vi "Main.vi"(7 "sweep rate, /min":dbl=0.2, 8 "sweep to:":dbl=-0.5, 9 "sweep":T6(radio)=enum."time_sweep") -> ()   [LabVIEW 2017] (continued)
                          tunnel: w749 -> [w752 w758]
                          tunnel: [w752 w757] -> w748
                          tunnel: w747 -> [w751 w755]
                          tunnel: [w751 w753] -> w746
                          frame False {
                            # "not measure 2182A 1 channel 1 (2182A_1_ch1)"
                          }
                          frame True {
                            w754 = "2182A_1_ch1"
                            # "measure 2182A 1 channel 1 (2182A_1_ch1)"
                            n675 = local read "2182A 1 addr"() -> (w759:u8)
                            n676 = Number To Decimal String(number=w759) -> (decimal integer string=w760:string)  [unwired: 1 in]
                            n677 = GPIB Clear(3:w760) -> ()  [unwired: 1 in, 2 out]
                            n678 = Build Array (concatenate)(w755, w754) -> (w753:string[])
                            n679 = Concatenate Strings(w758, w754, "\t") -> (w757:string)
                          }
                        }
                        n680 = property on="Figure_axis" class="Arr (strict)"("Value"=w746) -> ()  [unwired: 2 in, 2 out]
                        n681 = property on="data_caption" class="Str"("Value"=w748) -> ()  [unwired: 2 in, 2 out]
                      }
                      frame #27 {
                        # "2182A 1 channel 2 measure (2182A_1_ch2)"
                        n682 = local read "2182A 1 ch2"() -> (w765:bool)
                        n683 = property on="Figure_axis" class="Arr (strict)"() -> ("Value"=w762:string[])  [unwired: 2 in, 2 out]
                        n684 = property on="data_caption" class="Str"() -> ("Value"=w764:string)  [unwired: 2 in, 2 out]
                        n685 = case shown="True" w765 {
                          tunnel: w764 -> [w767 w773]
                          tunnel: [w767 w772] -> w763
                          tunnel: w762 -> [w766 w770]
                          tunnel: [w766 w768] -> w761
                          frame False {
                            # "not measure 2182A 1 channel 2 (2182A_1_ch2)"
                          }
                          frame True {
                            w769 = "2182A_1_ch2"
                            # "measure 2182A 1 channel 2 (2182A_1_ch2)"
                            n686 = local read "2182A 1 addr"() -> (w774:u8)
                            n687 = Number To Decimal String(number=w774) -> (decimal integer string=w775:string)  [unwired: 1 in]
                            n688 = GPIB Clear(3:w775) -> ()  [unwired: 1 in, 2 out]
                            n689 = Build Array (concatenate)(w770, w769) -> (w768:string[])
                            n690 = Concatenate Strings(w773, w769, "\t") -> (w772:string)
                          }
                        }
                        n691 = property on="Figure_axis" class="Arr (strict)"("Value"=w761) -> ()  [unwired: 2 in, 2 out]
                        n692 = property on="data_caption" class="Str"("Value"=w763) -> ()  [unwired: 2 in, 2 out]
                      }
                      frame #28 {
                        # "2182A 2 channel 1 measure (2182A_2_ch1)"
                        n693 = local read "2182A 2 ch1"() -> (w780:bool)
                        n694 = property on="Figure_axis" class="Arr (strict)"() -> ("Value"=w777:string[])  [unwired: 2 in, 2 out]
                        n695 = property on="data_caption" class="Str"() -> ("Value"=w779:string)  [unwired: 2 in, 2 out]
                        n696 = case shown="True" w780 {
                          tunnel: w779 -> [w782 w788]
                          tunnel: [w782 w787] -> w778
                          tunnel: w777 -> [w781 w785]
                          tunnel: [w781 w783] -> w776
                          frame False {
                            # "not measure 2182A 2 channel 1 (2182A_2_ch1)"
                          }
                          frame True {
                            w784 = "2182A_2_ch1"
                            # "measure 2182A 2 channel 1 (2182A_2_ch1)"
                            n697 = local read "2182A 2 addr"() -> (w789:u8)
                            n698 = Number To Decimal String(number=w789) -> (decimal integer string=w790:string)  [unwired: 1 in]
                            n699 = GPIB Clear(3:w790) -> ()  [unwired: 1 in, 2 out]
                            n700 = Build Array (concatenate)(w785, w784) -> (w783:string[])
                            n701 = Concatenate Strings(w788, w784, "\t") -> (w787:string)
                          }
                        }
                        n702 = property on="Figure_axis" class="Arr (strict)"("Value"=w776) -> ()  [unwired: 2 in, 2 out]
                        n703 = property on="data_caption" class="Str"("Value"=w778) -> ()  [unwired: 2 in, 2 out]
                      }
                      frame #29 {
                        # "2182A 2 channel 2 measure (2182A_2_ch2)"
                        n704 = local read "2182A 2 ch2"() -> (w795:bool)
                        n705 = property on="Figure_axis" class="Arr (strict)"() -> ("Value"=w792:string[])  [unwired: 2 in, 2 out]
                        n706 = property on="data_caption" class="Str"() -> ("Value"=w794:string)  [unwired: 2 in, 2 out]
                        n707 = case shown="True" w795 {
                          tunnel: w794 -> [w797 w803]
                          tunnel: [w797 w802] -> w793
                          tunnel: w792 -> [w796 w800]
                          tunnel: [w796 w798] -> w791
                          frame False {
                            # "not measure 2182A 2 channel 2 (2182A_2_ch2)"
                          }
                          frame True {
                            w799 = "2182A_2_ch2"
                            # "measure 2182A 2 channel 2 (2182A_2_ch2)"
                            n708 = local read "2182A 2 addr"() -> (w804:u8)
                            n709 = Number To Decimal String(number=w804) -> (decimal integer string=w805:string)  [unwired: 1 in]
                            n710 = GPIB Clear(3:w805) -> ()  [unwired: 1 in, 2 out]
                            n711 = Build Array (concatenate)(w800, w799) -> (w798:string[])
                            n712 = Concatenate Strings(w803, w799, "\t") -> (w802:string)
                          }
                        }
                        n713 = property on="Figure_axis" class="Arr (strict)"("Value"=w791) -> ()  [unwired: 2 in, 2 out]
                        n714 = property on="data_caption" class="Str"("Value"=w793) -> ()  [unwired: 2 in, 2 out]
                      }
                      frame #30 {
                        # "2182A 3 channel 1 measure (2182A_3_ch1)"
                        n715 = local read "2182A 3 ch1"() -> (w810:bool)
                        n716 = property on="Figure_axis" class="Arr (strict)"() -> ("Value"=w807:string[])  [unwired: 2 in, 2 out]
                        n717 = property on="data_caption" class="Str"() -> ("Value"=w809:string)  [unwired: 2 in, 2 out]
                        n718 = case shown="True" w810 {
                          tunnel: w809 -> [w812 w818]
                          tunnel: [w812 w817] -> w808
                          tunnel: w807 -> [w811 w815]
                          tunnel: [w811 w813] -> w806
                          frame False {
                            # "not measure 2182A 3 channel 1 (2182A_3_ch1)"
                          }
                          frame True {
                            w814 = "2182A_3_ch1"
                            # "measure 2182A 3 channel 1 (2182A_3_ch1)"
                            n719 = local read "2182A 3 addr"() -> (w819:u8)
                            n720 = Number To Decimal String(number=w819) -> (decimal integer string=w820:string)  [unwired: 1 in]
                            n721 = GPIB Clear(3:w820) -> ()  [unwired: 1 in, 2 out]
                            n722 = Build Array (concatenate)(w815, w814) -> (w813:string[])
                            n723 = Concatenate Strings(w818, w814, "\t") -> (w817:string)
                          }
                        }
                        n724 = property on="Figure_axis" class="Arr (strict)"("Value"=w806) -> ()  [unwired: 2 in, 2 out]
                        n725 = property on="data_caption" class="Str"("Value"=w808) -> ()  [unwired: 2 in, 2 out]
                      }
                      frame #31 {
                        # "2182A 3 channel 2 measure (2182A_3_ch2)"
                        n726 = local read "2182A 3 ch2"() -> (w825:bool)
                        n727 = property on="Figure_axis" class="Arr (strict)"() -> ("Value"=w822:string[])  [unwired: 2 in, 2 out]
                        n728 = property on="data_caption" class="Str"() -> ("Value"=w824:string)  [unwired: 2 in, 2 out]
                        n729 = case shown="False" w825 {
                          tunnel: w824 -> [w827 w833]
                          tunnel: [w827 w832] -> w823
                          tunnel: w822 -> [w826 w830]
                          tunnel: [w826 w828] -> w821
                          frame False {
                            # "not measure 2182A 3 channel 2 (2182A_3_ch2)"
                          }
                          frame True {
                            w829 = "2182A_3_ch2"
                            # "measure 2182A 3 channel 2 (2182A_3_ch2)"
                            n730 = local read "2182A 3 addr"() -> (w834:u8)
                            n731 = Number To Decimal String(number=w834) -> (decimal integer string=w835:string)  [unwired: 1 in]
                            n732 = GPIB Clear(3:w835) -> ()  [unwired: 1 in, 2 out]
                            n733 = Build Array (concatenate)(w830, w829) -> (w828:string[])
                            n734 = Concatenate Strings(w833, w829, "\t") -> (w832:string)
                          }
                        }
                        n735 = property on="Figure_axis" class="Arr (strict)"("Value"=w821) -> ()  [unwired: 2 in, 2 out]
                        n736 = property on="data_caption" class="Str"("Value"=w823) -> ()  [unwired: 2 in, 2 out]
                      }
                      frame #32 {
                        # "2182A 4 channel 1 measure (2182A_4_ch1)"
                        n737 = local read "2182A 4 ch1"() -> (w840:bool)
                        n738 = property on="Figure_axis" class="Arr (strict)"() -> ("Value"=w837:string[])  [unwired: 2 in, 2 out]
                        n739 = property on="data_caption" class="Str"() -> ("Value"=w839:string)  [unwired: 2 in, 2 out]
                        n740 = case shown="True" w840 {
                          tunnel: w839 -> [w842 w848]
                          tunnel: [w842 w847] -> w838
                          tunnel: w837 -> [w841 w845]
                          tunnel: [w841 w843] -> w836
                          frame False {
                            # "not measure 2182A 4 channel 1 (2182A_4_ch1)"
                          }
                          frame True {
                            w844 = "2182A_4_ch1"
                            # "measure 2182A 4 channel 1 (2182A_4_ch1)"
                            n741 = local read "2182A 4 addr"() -> (w849:u8)
                            n742 = Number To Decimal String(number=w849) -> (decimal integer string=w850:string)  [unwired: 1 in]
                            n743 = GPIB Clear(3:w850) -> ()  [unwired: 1 in, 2 out]
                            n744 = Build Array (concatenate)(w845, w844) -> (w843:string[])
                            n745 = Concatenate Strings(w848, w844, "\t") -> (w847:string)
                          }
                        }
                        n746 = property on="Figure_axis" class="Arr (strict)"("Value"=w836) -> ()  [unwired: 2 in, 2 out]
                        n747 = property on="data_caption" class="Str"("Value"=w838) -> ()  [unwired: 2 in, 2 out]
                      }
                      frame #33 {
                        # "2182A 4 channel 2 measure (2182A_4_ch2)"
                        n748 = local read "2182A 4 ch2"() -> (w855:bool)
                        n749 = property on="Figure_axis" class="Arr (strict)"() -> ("Value"=w852:string[])  [unwired: 2 in, 2 out]
                        n750 = property on="data_caption" class="Str"() -> ("Value"=w854:string)  [unwired: 2 in, 2 out]
                        n751 = case shown="True" w855 {
                          tunnel: w854 -> [w857 w863]
                          tunnel: [w857 w862] -> w853
                          tunnel: w852 -> [w856 w860]
                          tunnel: [w856 w858] -> w851
                          frame False {
                            # "not measure 2182A 4 channel 2 (2182A_4_ch2)"
                          }
                          frame True {
                            w859 = "2182A_4_ch2"
                            # "measure 2182A 4 channel 2 (2182A_4_ch2)"
                            n752 = local read "2182A 4 addr"() -> (w864:u8)
                            n753 = Number To Decimal String(number=w864) -> (decimal integer string=w865:string)  [unwired: 1 in]
                            n754 = GPIB Clear(3:w865) -> ()  [unwired: 1 in, 2 out]
                            n755 = Build Array (concatenate)(w860, w859) -> (w858:string[])
                            n756 = Concatenate Strings(w863, w859, "\t") -> (w862:string)
                          }
                        }
                        n757 = property on="Figure_axis" class="Arr (strict)"("Value"=w851) -> ()  [unwired: 2 in, 2 out]
                        n758 = property on="data_caption" class="Str"("Value"=w853) -> ()  [unwired: 2 in, 2 out]
                      }
                      frame #34 {
                        # "2636A smua measure voltage (2636A_smua_v)"
                        n759 = local read "2636A smua meas v"() -> (w870:bool)
                        n760 = property on="Figure_axis" class="Arr (strict)"() -> ("Value"=w867:string[])  [unwired: 2 in, 2 out]
                        n761 = property on="data_caption" class="Str"() -> ("Value"=w869:string)  [unwired: 2 in, 2 out]
                        n762 = case shown="True" w870 {
                          tunnel: w869 -> [w872 w883]
                          tunnel: [w872 w882] -> w868
                          tunnel: w867 -> [w871 w880]
                          tunnel: [w871 w878] -> w866
                          frame False {
                            # "not measure voltage on 2636A smua (2636A_smua_v)"
                          }
                          frame True {
                            w879 = "2636A_smua_v"
                            # "measure voltage on 2636A smua (2636A_smua_v)"
                            n763 = local read "2336A addr"() -> (w874:refnum<visa-resource-name>)
                            n764 = VISA Open(VISA resource name=w874) -> (VISA resource name=w873:refnum<visa-resource-name>, error out=w875:errorcluster)  [unwired: 4 in]
                            n765 = VISA Clear(VISA resource name=w873, error in (no error)=w875) -> (VISA resource name out=w877:refnum<visa-resource-name>)  [unwired: 1 out]
                            n766 = property class="Instr"(reference=w877, "General Settings:Timeout Value"=u32 10000) -> ()  [unwired: 1 in, 2 out]
                            n767 = Build Array (concatenate)(w880, w879) -> (w878:string[])
                            n768 = Concatenate Strings(w883, w879, "\t") -> (w882:string)
                          }
                        }
                        n769 = property on="Figure_axis" class="Arr (strict)"("Value"=w866) -> ()  [unwired: 2 in, 2 out]
                        n770 = property on="data_caption" class="Str"("Value"=w868) -> ()  [unwired: 2 in, 2 out]
                      }
                      frame #35 {
                        # "2636A smua measure current (2636A_smua_i)"
                        n771 = local read "2636A smua meas i"() -> (w888:bool)
                        n772 = property on="Figure_axis" class="Arr (strict)"() -> ("Value"=w885:string[])  [unwired: 2 in, 2 out]
                        n773 = property on="data_caption" class="Str"() -> ("Value"=w887:string)  [unwired: 2 in, 2 out]
                        n774 = case shown="True" w888 {
                          tunnel: w887 -> [w890 w901]
                          tunnel: [w890 w900] -> w886
                          tunnel: w885 -> [w889 w898]
                          tunnel: [w889 w896] -> w884
                          frame False {
                            # "not measure current on 2636A smua (2636A_smua_i)"
                          }
                          frame True {
                            w897 = "2636A_smua_i"
                            # "measure current on 2636A smua (2636A_smua_i)"
                            n775 = local read "2336A addr"() -> (w893:refnum<visa-resource-name>)
                            n776 = VISA Open(VISA resource name=w893) -> (VISA resource name=w892:refnum<visa-resource-name>, error out=w891:errorcluster)  [unwired: 4 in]
                            n777 = VISA Clear(VISA resource name=w892, error in (no error)=w891) -> (VISA resource name out=w894:refnum<visa-resource-name>)  [unwired: 1 out]
                            n778 = Build Array (concatenate)(w898, w897) -> (w896:string[])
                            n779 = property class="Instr"(reference=w894, "General Settings:Timeout Value"=u32 10000) -> ()  [unwired: 1 in, 2 out]
                            n780 = Concatenate Strings(w901, w897, "\t") -> (w900:string)
                          }
                        }
                        n781 = property on="Figure_axis" class="Arr (strict)"("Value"=w884) -> ()  [unwired: 2 in, 2 out]
                        n782 = property on="data_caption" class="Str"("Value"=w886) -> ()  [unwired: 2 in, 2 out]
                      }
                      frame #36 {
                        # "2636A smub measure voltage (2636A_smub_v)"
                        n783 = local read "2636A smub meas v"() -> (w906:bool)
                        n784 = property on="Figure_axis" class="Arr (strict)"() -> ("Value"=w903:string[])  [unwired: 2 in, 2 out]
                        n785 = property on="data_caption" class="Str"() -> ("Value"=w905:string)  [unwired: 2 in, 2 out]
                        n786 = case shown="True" w906 {
                          tunnel: w905 -> [w908 w919]
                          tunnel: [w908 w918] -> w904
                          tunnel: w903 -> [w907 w916]
                          tunnel: [w907 w914] -> w902
                          frame False {
                            # "not measure voltage on 2636A smub (2636A_smub_v)"
                          }
                          frame True {
                            w915 = "2636A_smub_v"
                            # "measure voltage on 2636A smub (2636A_smub_v)"
                            n787 = local read "2336A addr"() -> (w910:refnum<visa-resource-name>)
                            n788 = VISA Open(VISA resource name=w910) -> (VISA resource name=w909:refnum<visa-resource-name>, error out=w911:errorcluster)  [unwired: 4 in]
                            n789 = VISA Clear(VISA resource name=w909, error in (no error)=w911) -> (VISA resource name out=w912:refnum<visa-resource-name>)  [unwired: 1 out]
                            n790 = Build Array (concatenate)(w916, w915) -> (w914:string[])
                            n791 = property class="Instr"(reference=w912, "General Settings:Timeout Value"=u32 10000) -> ()  [unwired: 1 in, 2 out]
                            n792 = Concatenate Strings(w919, w915, "\t") -> (w918:string)
                          }
                        }
                        n793 = property on="Figure_axis" class="Arr (strict)"("Value"=w902) -> ()  [unwired: 2 in, 2 out]
                        n794 = property on="data_caption" class="Str"("Value"=w904) -> ()  [unwired: 2 in, 2 out]
                      }
                      frame #37 {
                        # "2636A smub measure current (2636A_smub_i)"
                        n795 = local read "2636A smub meas i"() -> (w924:bool)
                        n796 = property on="Figure_axis" class="Arr (strict)"() -> ("Value"=w921:string[])  [unwired: 2 in, 2 out]
                        n797 = property on="data_caption" class="Str"() -> ("Value"=w923:string)  [unwired: 2 in, 2 out]
                        n798 = case shown="True" w924 {
                          tunnel: w923 -> [w926 w937]
                          tunnel: [w926 w936] -> w922
                          tunnel: w921 -> [w925 w934]
                          tunnel: [w925 w932] -> w920
                          frame False {
                            # "not measure current on 2636A smub (2636A_smub_i)"
                          }
                          frame True {
                            w933 = "2636A_smub_i"
                            # "measure current on 2636A smub (2636A_smub_i)"
                            n799 = local read "2336A addr"() -> (w927:refnum<visa-resource-name>)
                            n800 = VISA Open(VISA resource name=w927) -> (VISA resource name=w928:refnum<visa-resource-name>, error out=w929:errorcluster)  [unwired: 4 in]
                            n801 = VISA Clear(VISA resource name=w928, error in (no error)=w929) -> (VISA resource name out=w930:refnum<visa-resource-name>)  [unwired: 1 out]
                            n802 = Build Array (concatenate)(w934, w933) -> (w932:string[])
                            n803 = property class="Instr"(reference=w930, "General Settings:Timeout Value"=u32 10000) -> ()  [unwired: 1 in, 2 out]
                            n804 = Concatenate Strings(w937, w933, "\t") -> (w936:string)
                          }
                        }
                        n805 = property on="Figure_axis" class="Arr (strict)"("Value"=w920) -> ()  [unwired: 2 in, 2 out]
                        n806 = property on="data_caption" class="Str"("Value"=w922) -> ()  [unwired: 2 in, 2 out]
                      }
                      frame #38 {
                        # "measure time"
                        n807 = local read "measure time"() -> (w942:bool)
                        n808 = property on="Figure_axis" class="Arr (strict)"() -> ("Value"=w939:string[])  [unwired: 2 in, 2 out]
                        n809 = property on="data_caption" class="Str"() -> ("Value"=w941:string)  [unwired: 2 in, 2 out]
                        n810 = case shown="True" w942 {
                          tunnel: w941 -> [w944 w950]
                          tunnel: [w944 w949] -> w940
                          tunnel: w939 -> [w943 w947]
                          tunnel: [w943 w945] -> w938
                          frame False {
                            # "not measuring time"
                          }
                          frame True {
                            w946 = "time"
                            # "measuring time"
                            n811 = Build Array (concatenate)(w947, w946) -> (w945:string[])
                            n812 = Concatenate Strings(w950, w946, "\t") -> (w949:string)
                          }
                        }
                        n813 = property on="Figure_axis" class="Arr (strict)"("Value"=w938) -> ()  [unwired: 2 in, 2 out]
                        n814 = property on="data_caption" class="Str"("Value"=w940) -> ()  [unwired: 2 in, 2 out]
                      }
                      frame #39 {
                        # "Measure magnetic field on IPS120-0"
                        n815 = local read "iPS_MagnetField"() -> (w955:bool)
                        n816 = property on="Figure_axis" class="Arr (strict)"() -> ("Value"=w952:string[])  [unwired: 2 in, 2 out]
                        n817 = property on="data_caption" class="Str"() -> ("Value"=w954:string)  [unwired: 2 in, 2 out]
                        n818 = case shown="True" w955 {
                          tunnel: w954 -> [w957 w963]
                          tunnel: [w957 w962] -> w953
                          tunnel: w952 -> [w956 w960]
                          tunnel: [w956 w958] -> w951
                          frame False {
                            # "do not Measure magnetic field on IPS120-0"
                          }
                          frame True {
                            w959 = "iPS_MagntField"
                            n819 = Build Array (concatenate)(w960, w959) -> (w958:string[])
                            n820 = Concatenate Strings(w963, w959, "\t") -> (w962:string)
                          }
                        }
                        n821 = property on="Figure_axis" class="Arr (strict)"("Value"=w951) -> ()  [unwired: 2 in, 2 out]
                        n822 = property on="data_caption" class="Str"("Value"=w953) -> ()  [unwired: 2 in, 2 out]
                      }
                      frame #40 {
                        # "Measure Magnet_T on iPS"
                        n823 = property on="Magnet_T" class="Bool (strict)"() -> ("Value"=w964:bool)  [unwired: 2 in, 2 out]
                        n824 = property on="Figure_axis" class="Arr (strict)"() -> ("Value"=w966:string[])  [unwired: 2 in, 2 out]
                        n825 = property on="data_caption" class="Str"() -> ("Value"=w968:string)  [unwired: 2 in, 2 out]
                        n826 = case shown="True" w964 {
                          tunnel: w968 -> [w970 w976]
                          tunnel: [w970 w975] -> w967
                          tunnel: w966 -> [w969 w973]
                          tunnel: [w969 w971] -> w965
                          frame False {
                            # "do not Measure magnetic field on IPS120-0"
                          }
                          frame True {
                            w972 = "iPS_Magnet_T"
                            n827 = Build Array (concatenate)(w973, w972) -> (w971:string[])
                            n828 = Concatenate Strings(w976, w972, "\t") -> (w975:string)
                          }
                        }
                        n829 = property on="Figure_axis" class="Arr (strict)"("Value"=w965) -> ()  [unwired: 2 in, 2 out]
                        n830 = property on="data_caption" class="Str"("Value"=w967) -> ()  [unwired: 2 in, 2 out]
                      }
                      frame #41 {
                        # "Measure SH_T on iPS"
                        n831 = property on="SH_T" class="Bool (strict)"() -> ("Value"=w977:bool)  [unwired: 2 in, 2 out]
                        n832 = property on="Figure_axis" class="Arr (strict)"() -> ("Value"=w979:string[])  [unwired: 2 in, 2 out]
                        n833 = property on="data_caption" class="Str"() -> ("Value"=w981:string)  [unwired: 2 in, 2 out]
                        n834 = case shown="False" w977 {
                          tunnel: w981 -> [w983 w989]
                          tunnel: [w983 w988] -> w980
                          tunnel: w979 -> [w982 w986]
                          tunnel: [w982 w984] -> w978
                          frame False {
                            # "do not Measure magnetic field on IPS120-0"
                          }
                          frame True {
                            w985 = "iPS_SH_T"
                            n835 = Build Array (concatenate)(w986, w985) -> (w984:string[])
                            n836 = Concatenate Strings(w989, w985, "\t") -> (w988:string)
                          }
                        }
                        n837 = property on="Figure_axis" class="Arr (strict)"("Value"=w978) -> ()  [unwired: 2 in, 2 out]
                        n838 = property on="data_caption" class="Str"("Value"=w980) -> ()  [unwired: 2 in, 2 out]
                      }
                      frame #42 {
                        # "iTC sample Temp"
                        n839 = property on="iTC_Sample_T" class="Bool (strict)"() -> ("Value"=w990:bool)  [unwired: 2 in, 2 out]
                        n840 = property on="Figure_axis" class="Arr (strict)"() -> ("Value"=w992:string[])  [unwired: 2 in, 2 out]
                        n841 = property on="data_caption" class="Str"() -> ("Value"=w994:string)  [unwired: 2 in, 2 out]
                        n842 = case shown="True" w990 {
                          tunnel: w994 -> [w996 w1002]
                          tunnel: [w996 w1001] -> w993
                          tunnel: w992 -> [w995 w999]
                          tunnel: [w995 w997] -> w991
                          frame False {
                            # "not measure 2461 voltage (2461_meas_v)"
                          }
                          frame True {
                            w998 = "iTC_Sample_T"
                            n843 = Build Array (concatenate)(w999, w998) -> (w997:string[])
                            n844 = Concatenate Strings(w1002, w998, "\t") -> (w1001:string)
                          }
                        }
                        n845 = property on="Figure_axis" class="Arr (strict)"("Value"=w991) -> ()  [unwired: 2 in, 2 out]
                        n846 = property on="data_caption" class="Str"("Value"=w993) -> ()  [unwired: 2 in, 2 out]
                      }
                      frame #43 {
                        # "iTC sample Temp"
                        n847 = property on="VTI_T" class="Bool (strict)"() -> ("Value"=w1003:bool)  [unwired: 2 in, 2 out]
                        n848 = property on="Figure_axis" class="Arr (strict)"() -> ("Value"=w1005:string[])  [unwired: 2 in, 2 out]
                        n849 = property on="data_caption" class="Str"() -> ("Value"=w1007:string)  [unwired: 2 in, 2 out]
                        n850 = case shown="True" w1003 {
                          tunnel: w1007 -> [w1009 w1015]
                          tunnel: [w1009 w1014] -> w1006
                          tunnel: w1005 -> [w1008 w1012]
                          tunnel: [w1008 w1010] -> w1004
                          frame False {
                            # "not measure 2461 voltage (2461_meas_v)"
                          }
                          frame True {
                            w1011 = "iTC_VTI_T"
                            n851 = Build Array (concatenate)(w1012, w1011) -> (w1010:string[])
                            n852 = Concatenate Strings(w1015, w1011, "\t") -> (w1014:string)
                          }
                        }
                        n853 = property on="Figure_axis" class="Arr (strict)"("Value"=w1004) -> ()  [unwired: 2 in, 2 out]
                        n854 = property on="data_caption" class="Str"("Value"=w1006) -> ()  [unwired: 2 in, 2 out]
                      }
                      frame #44 {
                        # "iTC sample Temp"
                        n855 = property on="PT1_T" class="Bool (strict)"() -> ("Value"=w1016:bool)  [unwired: 2 in, 2 out]
                        n856 = property on="Figure_axis" class="Arr (strict)"() -> ("Value"=w1018:string[])  [unwired: 2 in, 2 out]
                        n857 = property on="data_caption" class="Str"() -> ("Value"=w1020:string)  [unwired: 2 in, 2 out]
                        n858 = case shown="True" w1016 {
                          tunnel: w1020 -> [w1022 w1028]
                          tunnel: [w1022 w1027] -> w1019
                          tunnel: w1018 -> [w1021 w1025]
                          tunnel: [w1021 w1023] -> w1017
                          frame False {
                            # "not measure 2461 voltage (2461_meas_v)"
                          }
                          frame True {
                            w1024 = "iTC_PT1_T"
                            n859 = Build Array (concatenate)(w1025, w1024) -> (w1023:string[])
                            n860 = Concatenate Strings(w1028, w1024, "\t") -> (w1027:string)
                          }
                        }
                        n861 = property on="Figure_axis" class="Arr (strict)"("Value"=w1017) -> ()  [unwired: 2 in, 2 out]
                        n862 = property on="data_caption" class="Str"("Value"=w1019) -> ()  [unwired: 2 in, 2 out]
                      }
                      frame #45 {
                        # "iTC sample Temp"
                        n863 = property on="PT2_T" class="Bool (strict)"() -> ("Value"=w1029:bool)  [unwired: 2 in, 2 out]
                        n864 = property on="Figure_axis" class="Arr (strict)"() -> ("Value"=w1031:string[])  [unwired: 2 in, 2 out]
                        n865 = property on="data_caption" class="Str"() -> ("Value"=w1033:string)  [unwired: 2 in, 2 out]
                        n866 = case shown="True" w1029 {
                          tunnel: w1033 -> [w1035 w1041]
                          tunnel: [w1035 w1040] -> w1032
                          tunnel: w1031 -> [w1034 w1038]
                          tunnel: [w1034 w1036] -> w1030
                          frame False {
                            # "not measure 2461 voltage (2461_meas_v)"
                          }
                          frame True {
                            w1037 = "iTC_PT2_T"
                            n867 = Build Array (concatenate)(w1038, w1037) -> (w1036:string[])
                            n868 = Concatenate Strings(w1041, w1037, "\t") -> (w1040:string)
                          }
                        }
                        n869 = property on="Figure_axis" class="Arr (strict)"("Value"=w1030) -> ()  [unwired: 2 in, 2 out]
                        n870 = property on="data_caption" class="Str"("Value"=w1032) -> ()  [unwired: 2 in, 2 out]
                      }
                      frame #46 {
                        # "iTC sample Temp"
                        n871 = property on="VTI_P" class="Bool (strict)"() -> ("Value"=w1042:bool)  [unwired: 2 in, 2 out]
                        n872 = property on="Figure_axis" class="Arr (strict)"() -> ("Value"=w1044:string[])  [unwired: 2 in, 2 out]
                        n873 = property on="data_caption" class="Str"() -> ("Value"=w1046:string)  [unwired: 2 in, 2 out]
                        n874 = case shown="True" w1042 {
                          tunnel: w1046 -> [w1048 w1054]
                          tunnel: [w1048 w1053] -> w1045
                          tunnel: w1044 -> [w1047 w1051]
                          tunnel: [w1047 w1049] -> w1043
                          frame False {
                            # "not measure 2461 voltage (2461_meas_v)"
                          }
                          frame True {
                            w1050 = "iTC_VTI_P"
                            n875 = Build Array (concatenate)(w1051, w1050) -> (w1049:string[])
                            n876 = Concatenate Strings(w1054, w1050, "\t") -> (w1053:string)
                          }
                        }
                        n877 = property on="Figure_axis" class="Arr (strict)"("Value"=w1043) -> ()  [unwired: 2 in, 2 out]
                        n878 = property on="data_caption" class="Str"("Value"=w1045) -> ()  [unwired: 2 in, 2 out]
                      }
                      frame #47 {
                        # "iTC sample Temp"
                        n879 = property on="2461_meas_v" class="Bool (strict)"() -> ("Value"=w1055:bool)  [unwired: 2 in, 2 out]
                        n880 = property on="Figure_axis" class="Arr (strict)"() -> ("Value"=w1057:string[])  [unwired: 2 in, 2 out]
                        n881 = property on="data_caption" class="Str"() -> ("Value"=w1059:string)  [unwired: 2 in, 2 out]
                        n882 = case shown="True" w1055 {
                          tunnel: w1059 -> [w1061 w1067]
                          tunnel: [w1061 w1066] -> w1058
                          tunnel: w1057 -> [w1060 w1064]
                          tunnel: [w1060 w1062] -> w1056
                          frame False {
                            # "not measure 2461 voltage (2461_meas_v)"
                          }
                          frame True {
                            w1063 = "2461_meas_v"
                            n883 = Build Array (concatenate)(w1064, w1063) -> (w1062:string[])
                            n884 = Concatenate Strings(w1067, w1063, "\t") -> (w1066:string)
                          }
                        }
                        n885 = property on="Figure_axis" class="Arr (strict)"("Value"=w1056) -> ()  [unwired: 2 in, 2 out]
                        n886 = property on="data_caption" class="Str"("Value"=w1058) -> ()  [unwired: 2 in, 2 out]
                      }
                      frame #48 {
                        # "iTC sample Temp"
                        n887 = property on="2461_meas_i" class="Bool (strict)"() -> ("Value"=w1068:bool)  [unwired: 2 in, 2 out]
                        n888 = property on="Figure_axis" class="Arr (strict)"() -> ("Value"=w1070:string[])  [unwired: 2 in, 2 out]
                        n889 = property on="data_caption" class="Str"() -> ("Value"=w1072:string)  [unwired: 2 in, 2 out]
                        n890 = case shown="True" w1068 {
                          tunnel: w1072 -> [w1074 w1080]
                          tunnel: [w1074 w1079] -> w1071
                          tunnel: w1070 -> [w1073 w1077]
                          tunnel: [w1073 w1075] -> w1069
                          frame False {
                            # "not measure 2461 voltage (2461_meas_v)"
                          }
                          frame True {
                            w1076 = "2461_meas_i"
                            n891 = Build Array (concatenate)(w1077, w1076) -> (w1075:string[])
                            n892 = Concatenate Strings(w1080, w1076, "\t") -> (w1079:string)
                          }
                        }
                        n893 = property on="Figure_axis" class="Arr (strict)"("Value"=w1069) -> ()  [unwired: 2 in, 2 out]
                        n894 = property on="data_caption" class="Str"("Value"=w1071) -> ()  [unwired: 2 in, 2 out]
                      }
                      frame #49 {
                        # "iTC sample Temp"
                        n895 = property on="Step Loop" class="Bool (strict)"() -> ("Value"=w1081:bool)  [unwired: 2 in, 2 out]
                        n896 = property on="Figure_axis" class="Arr (strict)"() -> ("Value"=w1083:string[])  [unwired: 2 in, 2 out]
                        n897 = property on="data_caption" class="Str"() -> ("Value"=w1085:string)  [unwired: 2 in, 2 out]
                        n898 = case shown="True" w1081 {
                          tunnel: w1085 -> [w1087 w1096]
                          tunnel: [w1087 w1095] -> w1084
                          tunnel: w1083 -> [w1086 w1093]
                          tunnel: [w1086 w1092] -> w1082
                          frame False {
                            # "not measure 2461 voltage (2461_meas_v)"
                          }
                          frame True {
                            n899 = property on="step" class="RadioBtnsControl (strict)"() -> ("Value"=w1091:T8)  [unwired: 2 in, 2 out]
                            n900 = case shown="\"iPS_step\"" w1091 {
                              tunnel: ["V2400_1" "V2400_2" "Va" "Vb" "time" "iTC" "iPS"] -> w1089
                              frame "V2400_1_Step", Default {
                              }
                              frame "V2400_2_step" {
                              }
                              frame "2636_smua_step" {
                              }
                              frame "2636_smub_step" {
                              }
                              frame "time_step" {
                              }
                              frame "iTC_step" {
                              }
                              frame "iPS_step" {
                              }
                            }
                            n901 = Concatenate Strings(w1089, "_Step") -> (w1088:string)
                            n902 = Build Array (concatenate)(w1093, w1088) -> (w1092:string[])
                            n903 = Concatenate Strings(w1096, w1088, "\t") -> (w1095:string)
                          }
                        }
                        n904 = property on="Figure_axis" class="Arr (strict)"("Value"=w1082) -> ()  [unwired: 2 in, 2 out]
                        n905 = property on="data_caption" class="Str"("Value"=w1084) -> ()  [unwired: 2 in, 2 out]
                      }
                      frame #50 {
                        # "iTC sample Temp"
                        n906 = property on="HyperLoop" class="Bool (strict)"() -> ("Value"=w1104:bool)  [unwired: 2 in, 2 out]
                        n907 = property on="Figure_axis" class="Arr (strict)"() -> ("Value"=w1106:string[])  [unwired: 2 in, 2 out]
                        n908 = property on="data_caption" class="Str"() -> ("Value"=w1108:string)  [unwired: 2 in, 2 out]
                        n909 = case shown="True" w1104 {
                          tunnel: w1108 -> [w1110 w1119]
                          tunnel: [w1110 w1118] -> w1107
                          tunnel: w1106 -> [w1109 w1116]
                          tunnel: [w1109 w1115] -> w1105
                          frame False {
                            # "not measure 2461 voltage (2461_meas_v)"
                          }
                          frame True {
                            n910 = property on="step_hyper" class="RadioBtnsControl (strict)"() -> ("Value"=w1114:T9)  [unwired: 2 in, 2 out]
                            n911 = case shown="\"iPS_HyperLoop\"" w1114 {
                              tunnel: ["V2400_1" "V2400_2" "Va" "Vb" "time" "iTC" "iPS"] -> w1112
                              frame "2400_1_HyperLoop", Default {
                              }
                              frame "2400_2_HyperLoop" {
                              }
                              frame "2636_smua_HyperLoop" {
                              }
                              frame "2636_smub_HyperLoop" {
                              }
                              frame "time_HyperLoop" {
                              }
                              frame "iTC_HyperLoop" {
                              }
                              frame "iPS_HyperLoop" {
                              }
                            }
                            n912 = Concatenate Strings(w1112, "_HyperLoop") -> (w1111:string)
                            n913 = Build Array (concatenate)(w1116, w1111) -> (w1115:string[])
                            n914 = Concatenate Strings(w1119, w1111, "\t") -> (w1118:string)
                          }
                        }
                        n915 = property on="Figure_axis" class="Arr (strict)"("Value"=w1105) -> ()  [unwired: 2 in, 2 out]
                        n916 = property on="data_caption" class="Str"("Value"=w1107) -> ()  [unwired: 2 in, 2 out]
                      }
                      frame #51 {
                        # "iTC sample Temp"
                        n917 = property on="SuperHyper" class="Bool (strict)"() -> ("Value"=w1127:bool)  [unwired: 2 in, 2 out]
                        n918 = property on="data_caption" class="Str"() -> ("Value"=w1131:string)  [unwired: 2 in, 2 out]
                        n919 = property on="Figure_axis" class="Arr (strict)"() -> ("Value"=w1129:string[])  [unwired: 2 in, 2 out]
                        n920 = case shown="True" w1127 {
                          tunnel: w1131 -> [w1133 w1142]
                          tunnel: [w1133 w1141] -> w1130
                          tunnel: w1129 -> [w1132 w1139]
                          tunnel: [w1132 w1138] -> w1128
                          frame False {
                            # "not measure 2461 voltage (2461_meas_v)"
                          }
                          frame True {
                            n921 = property on="step_super" class="RadioBtnsControl (strict)"() -> ("Value"=w1134:T10)  [unwired: 2 in, 2 out]
                            n922 = case shown="\"iTC_SuperHyper\"" w1134 {
                              tunnel: ["V2400_1" "V2400_2" "Va" "Vb" "time" "iTC" "iPS"] -> w1136
                              frame "2400_1_SuperHyper", Default {
                              }
                              frame "2400_2_SuperHyper" {
                              }
                              frame "2636_smua_SuperHyper" {
                              }
                              frame "2636_smub_SuperHyper" {
                              }
                              frame "time_SuperHyper" {
                              }
                              frame "iTC_SuperHyper" {
                              }
                              frame "iPS_SuperHyper" {
                              }
                            }
                            n923 = Concatenate Strings(w1136, "_SuperHyper") -> (w1135:string)
                            n924 = Build Array (concatenate)(w1139, w1135) -> (w1138:string[])
                            n925 = Concatenate Strings(w1142, w1135, "\t") -> (w1141:string)
                          }
                        }
                        n926 = property on="Figure_axis" class="Arr (strict)"("Value"=w1128) -> ()  [unwired: 2 in, 2 out]
                        n927 = property on="data_caption" class="Str"("Value"=w1130) -> ()  [unwired: 2 in, 2 out]
                      }
                    }
                  }
                  frame #2 {
                    # "0 = SR830_1_ip\n1 = SR830_1_oop\n2 = SR830_2_ip\n3 = SR830_2_oop\n4 = SR830_3_ip\n5 = SR830_3_oop\n6 = SR830_4_ip \n7 = SR830_4_oop \n8 = SR830_5_ip \n9 = SR830_5_oop \n10= 2400_1_v \n11= 2400_1_i \n12 = 2400_2_v\n13 = 2400_2_i \n14 = 2400_3_v \n15 = 2400_3_i \n16 = 2182A_1_ch1 \n17 = 2182A_1_ch2 \n18 = 2182A_2_ch1 \n19 = 2182A_2_ch2\n20 = 2182A_3_ch1 \n21 = 2182A_3_ch2 \n22 = 2182A_4_ch1 \n23 = 2182A_4_ch2 \n24 = 2636A_smua_v \n25 = 2636A_smua_i \n26 = 2636A_smub_v \n27 = 2636A_smub_i \n28 = time\n29 = iPS_Field\n30 = iPS_Magnet_T\n31 = iPS__SH_T\n32 = iTC _sample_T\n33 = iTC _VTI_T\n34 = iTC _PT1_T\n35 = iTC _PT2_T\n36 = iTC _VTI_P\n37 = 2461_meas_v\n38= 2461_meas_i\n39= Step_Value\n40= HyperLoop_Step\n41= SuperHyper_Step"
                    n928 = stacked-sequence {
                      frame #0 {
                        w1154 = dbl[] []  # Empty array for data
                        # "clear data array before each measurement cycle"
                        n929 = property on="data" class="Arr (strict)"("Value"=w1154) -> (error out=w1153:errorcluster)  [unwired: 2 in, 1 out]
                        n930 = property on="Sweep Channel" class="DigNum (strict)"() -> ("Value"=w1150:dbl)  [unwired: 2 in, 2 out]
                        n931 = property on="data" class="Arr (strict)"(error in=w1153) -> ("Value"=w1152:dbl[])  [unwired: 1 in, 2 out]
                        n932 = Build Array (concatenate)(w1152, w1150) -> (w1151:dbl[])
                        n933 = property on="data" class="Arr (strict)"("Value"=w1151) -> ()  [unwired: 2 in, 2 out]
                      }
                      frame #1 {
                        n934 = stacked-sequence "measurement sequence" {
                          frame #0 {
                            # "check if in-phase\nsignal on lock-in 1 \nis to be measured"
                            n935 = property on="data" class="Arr (strict)"() -> ("Value"=w1156:dbl[])  [unwired: 2 in, 2 out]
                            n936 = local read "SR830 1 ip"() -> (w1155:bool)
                            n937 = case shown="True" w1155 {
                              tunnel: w1156 -> [w1158 w1167]
                              tunnel: [w1158 w1166] -> w1157
                              frame False {
                                # "we are not measuring in phase signal on lock-in 1 (SR830_1_ip)"
                              }
                              frame True {
                                # "we are  measuring lock-in 1, in phase (SR830_1_ip)"
                                n938 = local read "SR830 1 addr"() -> (w1160:u8)
                                n939 = Number To Decimal String(number=w1160) -> (decimal integer string=w1159:string)  [unwired: 1 in]
                                n940 = GPIB Write(0:w1159, 1:"OUTR?1") -> (6:w1165:errorcluster)  [unwired: 3 in, 1 out]
                                n941 = GPIB Read(0:w1159, 1:3200, 3:w1165) -> (5:w1163:string)  [unwired: 2 in, 2 out]
                                n942 = Fract/Exp String To Number(string=w1163) -> (number=w1162:dbl)  [unwired: 3 in, 1 out]
                                n943 = Build Array (concatenate)(w1167, w1162) -> (w1166:dbl[])
                              }
                            }
                            n944 = property on="data" class="Arr (strict)"("Value"=w1157) -> ()  [unwired: 2 in, 2 out]
                          }
                          frame #1 {
                            # "check if out-of-phase\nsignal on lock-in 1 \nis to be measured"
                            n945 = property on="data" class="Arr (strict)"() -> ("Value"=w1169:dbl[])  [unwired: 2 in, 2 out]
                            n946 = local read "SR830 1 oop"() -> (w1168:bool)
                            n947 = case shown="True" w1168 {
                              tunnel: w1169 -> [w1171 w1180]
                              tunnel: [w1171 w1179] -> w1170
                              frame False {
                                # "we are not measuring out of phase signal on lock-in 1 (SR830_1_oop)"
                              }
                              frame True {
                                # "we are  measuring lock-in 1, out of phase (SR830_1_oop)"
                                n948 = local read "SR830 1 addr"() -> (w1173:u8)
                                n949 = Number To Decimal String(number=w1173) -> (decimal integer string=w1172:string)  [unwired: 1 in]
                                n950 = GPIB Write(0:w1172, 1:"OUTR?2") -> (6:w1178:errorcluster)  [unwired: 3 in, 1 out]
                                n951 = GPIB Read(0:w1172, 1:3200, 3:w1178) -> (5:w1176:string)  [unwired: 2 in, 2 out]
                                n952 = Fract/Exp String To Number(string=w1176) -> (number=w1175:dbl)  [unwired: 3 in, 1 out]
                                n953 = Build Array (concatenate)(w1180, w1175) -> (w1179:dbl[])
                              }
                            }
                            n954 = property on="data" class="Arr (strict)"("Value"=w1170) -> ()  [unwired: 2 in, 2 out]
                          }
                          frame #2 {
                            # "check if in-phase\nsignal on lock-in 2 \nis to be measured"
                            n955 = property on="data" class="Arr (strict)"() -> ("Value"=w1182:dbl[])  [unwired: 2 in, 2 out]
                            n956 = local read "SR830 2 ip"() -> (w1181:bool)
                            n957 = case shown="True" w1181 {
                              tunnel: w1182 -> [w1184 w1193]
                              tunnel: [w1184 w1192] -> w1183
                              frame False {
                                # "we are not measuring in phase signal on lock-in 2 (SR830_2_ip)"
                              }
                              frame True {
                                # "we are  measuring lock-in 2, in phase (SR830_2_ip)"
                                n958 = local read "SR830 2 addr"() -> (w1186:u8)
                                n959 = Number To Decimal String(number=w1186) -> (decimal integer string=w1185:string)  [unwired: 1 in]
                                n960 = GPIB Write(0:w1185, 1:"OUTP?1") -> (6:w1191:errorcluster)  [unwired: 3 in, 1 out]
                                n961 = GPIB Read(0:w1185, 1:3200, 3:w1191) -> (5:w1189:string)  [unwired: 2 in, 2 out]
                                n962 = Fract/Exp String To Number(string=w1189) -> (number=w1188:dbl)  [unwired: 3 in, 1 out]
                                n963 = Build Array (concatenate)(w1193, w1188) -> (w1192:dbl[])
                              }
                            }
                            n964 = property on="data" class="Arr (strict)"("Value"=w1183) -> ()  [unwired: 2 in, 2 out]
                          }
                          frame #3 {
                            # "check if out-of-phase\nsignal on lock-in 2 \nis to be measured"
                            n965 = property on="data" class="Arr (strict)"() -> ("Value"=w1195:dbl[])  [unwired: 2 in, 2 out]
                            n966 = local read "SR830 2 oop"() -> (w1194:bool)
                            n967 = case shown="True" w1194 {
                              tunnel: w1195 -> [w1197 w1206]
                              tunnel: [w1197 w1205] -> w1196
                              frame False {
                                # "we are not measuring out of phase signal on lock-in 2 (SR830_2_oop)"
                              }
                              frame True {
                                # "we are  measuring lock-in 2, out of phase (SR830_2_oop)"
                                n968 = local read "SR830 2 addr"() -> (w1199:u8)
                                n969 = Number To Decimal String(number=w1199) -> (decimal integer string=w1198:string)  [unwired: 1 in]
                                n970 = GPIB Write(0:w1198, 1:"OUTP?2") -> (6:w1204:errorcluster)  [unwired: 3 in, 1 out]
                                n971 = GPIB Read(0:w1198, 1:3200, 3:w1204) -> (5:w1202:string)  [unwired: 2 in, 2 out]
                                n972 = Fract/Exp String To Number(string=w1202) -> (number=w1201:dbl)  [unwired: 3 in, 1 out]
                                n973 = Build Array (concatenate)(w1206, w1201) -> (w1205:dbl[])
                              }
                            }
                            n974 = property on="data" class="Arr (strict)"("Value"=w1196) -> ()  [unwired: 2 in, 2 out]
                          }
                          frame #4 {
                            # "check if in-phase\nsignal on lock-in 3 \nis to be measured"
                            n975 = property on="data" class="Arr (strict)"() -> ("Value"=w1208:dbl[])  [unwired: 2 in, 2 out]
                            n976 = local read "SR830 3 ip"() -> (w1207:bool)
                            n977 = case shown="True" w1207 {
                              tunnel: w1208 -> [w1210 w1219]
                              tunnel: [w1210 w1218] -> w1209
                              frame False {
                                # "we are not measuring in phase signal on lock-in 3 (SR830_3_ip)"
                              }
                              frame True {
                                # "we are  measuring lock-in 3, in phase (SR830_3_ip)"
                                n978 = local read "SR830 3 addr"() -> (w1212:u8)
                                n979 = Number To Decimal String(number=w1212) -> (decimal integer string=w1211:string)  [unwired: 1 in]
                                n980 = GPIB Write(0:w1211, 1:"OUTP?1") -> (6:w1217:errorcluster)  [unwired: 3 in, 1 out]
                                n981 = GPIB Read(0:w1211, 1:3200, 3:w1217) -> (5:w1215:string)  [unwired: 2 in, 2 out]
                                n982 = Fract/Exp String To Number(string=w1215) -> (number=w1214:dbl)  [unwired: 3 in, 1 out]
                                n983 = Build Array (concatenate)(w1219, w1214) -> (w1218:dbl[])
                              }
                            }
                            n984 = property on="data" class="Arr (strict)"("Value"=w1209) -> ()  [unwired: 2 in, 2 out]
                          }
                          frame #5 {
                            # "check if out-of-phase\nsignal on lock-in 3 \nis to be measured"
                            n985 = property on="data" class="Arr (strict)"() -> ("Value"=w1221:dbl[])  [unwired: 2 in, 2 out]
                            n986 = local read "SR830 3 oop"() -> (w1220:bool)
                            n987 = case shown="True" w1220 {
                              tunnel: w1221 -> [w1223 w1232]
                              tunnel: [w1223 w1231] -> w1222
                              frame False {
                                # "we are not measuring out of phase signal on lock-in 3 (SR830_3_oop)"
                              }
                              frame True {
                                # "we are  measuring lock-in 3, out of phase (SR830_3_oop)"
                                n988 = local read "SR830 3 addr"() -> (w1225:u8)
                                n989 = Number To Decimal String(number=w1225) -> (decimal integer string=w1224:string)  [unwired: 1 in]
                                n990 = GPIB Write(0:w1224, 1:"OUTP?2") -> (6:w1230:errorcluster)  [unwired: 3 in, 1 out]
                                n991 = GPIB Read(0:w1224, 1:3200, 3:w1230) -> (5:w1228:string)  [unwired: 2 in, 2 out]
                                n992 = Fract/Exp String To Number(string=w1228) -> (number=w1227:dbl)  [unwired: 3 in, 1 out]
                                n993 = Build Array (concatenate)(w1232, w1227) -> (w1231:dbl[])
                              }
                            }
                            n994 = property on="data" class="Arr (strict)"("Value"=w1222) -> ()  [unwired: 2 in, 2 out]
                          }
                          frame #6 {
                            # "check if in-phase\nsignal on lock-in 4 \nis to be measured"
                            n995 = property on="data" class="Arr (strict)"() -> ("Value"=w1234:dbl[])  [unwired: 2 in, 2 out]
                            n996 = local read "SR830 4 ip"() -> (w1233:bool)
                            n997 = case shown="True" w1233 {
                              tunnel: w1234 -> [w1236 w1245]
                              tunnel: [w1236 w1244] -> w1235
                              frame False {
                                # "we are not measuring in phase signal on lock-in 4 (SR830_4_ip)"
                              }
                              frame True {
                                # "we are  measuring lock-in 4, in phase (SR830_4_ip)"
                                n998 = local read "SR830 4 addr"() -> (w1238:u8)
                                n999 = Number To Decimal String(number=w1238) -> (decimal integer string=w1237:string)  [unwired: 1 in]
                                n1000 = GPIB Write(0:w1237, 1:"OUTP?1") -> (6:w1243:errorcluster)  [unwired: 3 in, 1 out]
                                n1001 = GPIB Read(0:w1237, 1:3200, 3:w1243) -> (5:w1241:string)  [unwired: 2 in, 2 out]
                                n1002 = Fract/Exp String To Number(string=w1241) -> (number=w1240:dbl)  [unwired: 3 in, 1 out]
                                n1003 = Build Array (concatenate)(w1245, w1240) -> (w1244:dbl[])
                              }
                            }
                            n1004 = property on="data" class="Arr (strict)"("Value"=w1235) -> ()  [unwired: 2 in, 2 out]
                          }
                          frame #7 {
                            # "check if out-of-phase\nsignal on lock-in 4 \nis to be measured"
                            n1005 = property on="data" class="Arr (strict)"() -> ("Value"=w1247:dbl[])  [unwired: 2 in, 2 out]
                            n1006 = local read "SR830 4 oop"() -> (w1246:bool)
                            n1007 = case shown="True" w1246 {
                              tunnel: w1247 -> [w1249 w1258]
                              tunnel: [w1249 w1257] -> w1248
                              frame False {
                                # "we are not measuring out of phase signal on lock-in 4 (SR830_4_oop)"
                              }
                              frame True {
                                # "we are  measuring lock-in 4, out of phase (SR830_4_oop)"
                                n1008 = local read "SR830 4 addr"() -> (w1251:u8)
